vi "Clear.vi"(8 "error in (no error)":errorcluster, 11 "Simulation Interface in":refnum<class "Simulation Interface.lvclass">) -> (0 "error out":errorcluster)   [LabVIEW 2016, in "Simulation Interface.lvclass"]
uses:
  Simulation Interface.lvclass
  Database/Database.lvclass
  Error Handler/Error Handler.lvclass
  Error Handler/EH Action.ctl
  Car Wash Controller/Car Wash Controller.lvclass
  Wash Display Console/Wash Display Console.lvclass
  Vehicle Position Simulation/Vehicle Position Simulation.lvclass
  Entry Console/Entry Console.lvclass
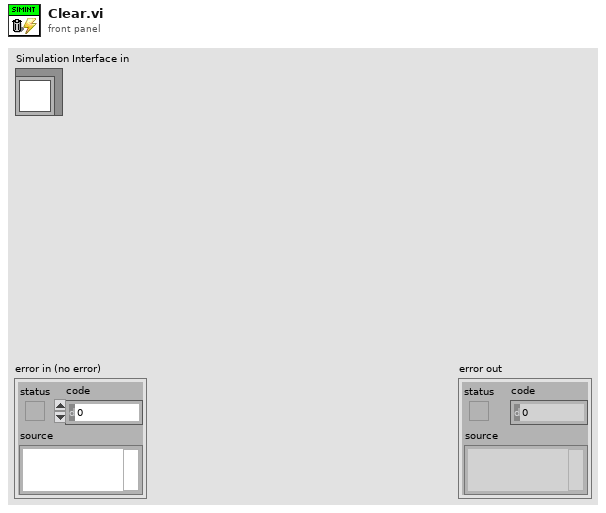
[diagram p1: front panel]
types:
  T1 = typedef "Architecture.lvlib/Error Handler.lvclass/EH Action.ctl" = enum16{"Define Threads", "Close", "System Error", "Wash Cycle Error", "Minor Error", "Initialize"}
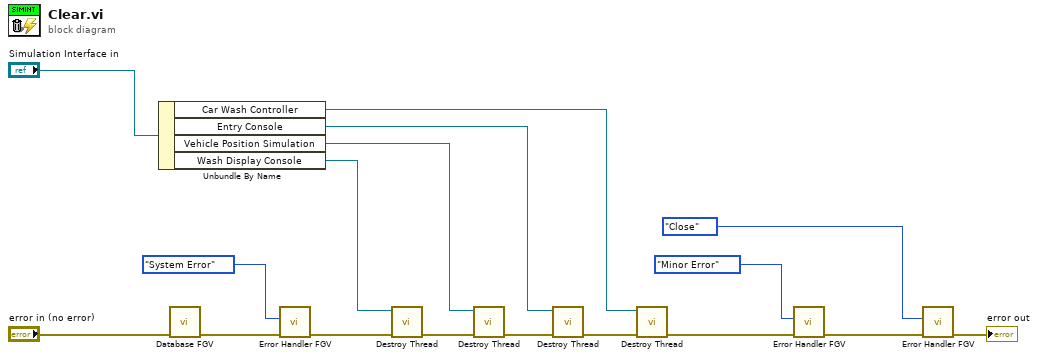
[diagram p0: block diagram]
diagram:
  n1 = Unbundle By Name("Simulation Interface in") -> ("Car Wash Controller"=w1:refnum<class "Car Wash Controller.lvclass">, "Entry Console"=w2:refnum<class "Entry Console.lvclass">, "Vehicle Position Simulation"=w3:refnum<class "Vehicle Position Simulation.lvclass">, "Wash Display Console"=w4:refnum<class "Wash Display Console.lvclass">)
  n2 = call "Database FGV.vi"("error in (no error)"="error in (no error)") -> ("error out"=w7:errorcluster)  [unwired: 8 in, 2 out]
  n3 = call "Error Handler FGV.vi"("error in (no error)"=w7, "Action"=EH_Action."System Error") -> ("error out"=w5:errorcluster)  [unwired: 9 in]
  n4 = call-dynamic "Destroy Thread.vi"("error in (no error)"=w5, "Thread in"=w4) -> ("error out"=w16:errorcluster)  [unwired: 9 in]
  n5 = call-dynamic "Destroy Thread.vi"("error in (no error)"=w16, "Thread in"=w3) -> ("error out"=w15:errorcluster)  [unwired: 9 in]
  n6 = call-dynamic "Destroy Thread.vi"("error in (no error)"=w15, "Thread in"=w2) -> ("error out"=w14:errorcluster)  [unwired: 9 in]
  n7 = call-dynamic "Destroy Thread.vi"("error in (no error)"=w14, "Thread in"=w1) -> ("error out"=w11:errorcluster)  [unwired: 9 in]
  n8 = call "Error Handler FGV.vi"("error in (no error)"=w11, "Action"=EH_Action."Minor Error") -> ("error out"=w10:errorcluster)  [unwired: 9 in]
  n9 = call "Error Handler FGV.vi"("error in (no error)"=w10, "Action"=EH_Action."Close") -> ("error out"=→"error out":errorcluster)  [unwired: 9 in]
